vi "ExampleAll64.vi"() -> ()   [LabVIEW 2009]
uses:
  <userlib>/Untitled 5 Folder/user.lib/Shamrock64.llb/shamrock_flipperPort_typedef.ctl
  <userlib>/Untitled 5 Folder/user.lib/Shamrock64.llb/shamrock_lipperMirror_typedef.ctl
panel:
  in  "Device":i32 min=0 max=1
  in  "Set Device":bool
  in  "Tab Control":T1(tab)
  in  "Grating Offset":i32
  out "SetGratingOffset":string
  in  "Detector Offset":i32
  out "SetDetectorOffset":string
  out "WavelengthReset":string
  out "SetGrating":string
  in  "Grating":i32
  in  "Turret":i32
  out "SetTurret":string
  in  "SetGratingOffset":bool
  in  "SetDetectorOffset":bool
  in  "WavelengthReset":bool
  in  "SetGrating":bool
  in  "SetTurret":bool
  out "blaze":string
  out "Grating Offset":i32
  out "Detector Offset":i32
  out "offset":i32
  out "home":i32
  out "lines/mm":dbl format="%.2f"
  out "Grating":i32
  out "No Gratings":i32
  out "Turret":i32
  out "Is Grating ?":string
  out "GetGratingOffset":string
  out "GetDetectorOffset":string
  out "GetGratingInfo":string
  out "GetGrating":string
  out "GetNumberGratings":string
  out "GetTurret":string
  out "GratingIsPresent":string
  out "GetCalibration":string
  out "SetNumberPixels":string
  out "SetPixelWidth":string
  out "Max Dispersion":sgl
  out "Min Dispersion":sgl
  in  "Number Pixels":u32 caption="Numeric"
  in  "Pixel Width":sgl caption="Numeric" format="%_3g"
  out "GotoZeroOrder":string
  out "SetWavelength":string
  in  "Wavelength":dbl format="%.2f"
  in  "GoToZeroOrder":bool
  out "Max Wavelength":dbl format="%.2f"
  out "Min Wavelength":dbl format="%.2f"
  out "Is Wavelength ?":string
  out "WavelengthIsPresent":string
  out "GetWavelengthLimits":string
  out "At Zero Order ?":string
  out "AtZeroOrder":string
  out "Wavelength":dbl format="%.2f"
  in  "SetWavelength 2":bool
  out "GetWavelength":string
  in  "Reset Output Slit":bool
  in  "Reset Slit":bool
  out "ResetOutputSlit":string
  out "ResetSlit":string
  out "SetOutputSlit":string
  out "SetSlit":string
  in  "Output Slit Width":dbl format="%.2f"
  in  "SetOuputSlit":bool
  in  "Slit Width":dbl format="%.2f"
  in  "SetSlit 2":bool
  out "Output Slit width(mm)":dbl format="%.2f"
  out "Slit width (mm)":dbl format="%.2f"
  out "Is Output Slit ?":string
  out "Is Input Slit ?":string
  out "GetOutputSlit":string
  out "GetSlit":string
  out "OutputSlitIsPresent":string
  out "SlitIsPresent":string
  in  "Mode":i32
  in  "SetShutter":bool
  out "Is Mode Possible ?":string
  out "Shutter":i32
  out "Is Shutter ?":string
  out "SetShutter":string
  out "IsModePossible":string
  out "GetShutter":string
  out "ShutterIsPresent":string
  in  "Flipper Port":T2
  out "High":dbl format="%.2f"
  in  "FlipperReset":bool
  out "FlipperReset":string
  in  "SetPort":bool
  out "Low":dbl format="%.2f"
  out "Port":T2
  out "Is Flipper ?":string
  out "SetPort":string
  out "GetCCDLimits":string
  out "GetPort":string
  out "FlipperIsPresent":string
  out "GetFlipperMirror":string
  in  "FlipperSelect":bool
  in  "Flipper Mirror":T3
  in  "Filter info":string caption="String"
  out "Filter Info":string
  in  "SetFilterInfo":bool
  out "SetFilterInfo":string
  in  "Filter":i32
  in  "SetFilter":bool
  out "Filter":i32
  out "Is Filter ?":string
  out "SetFilter":string
  out "GetFilterInfo":string
  out "GetFilter":string
  out "FilterIsPresent":string
  in  "Line":i32
  out "Line 2":i32
  in  "State":i32
  in  "Set Accessory":bool
  out "Line 1":i32
  out "Is Accessory ?":string
  out "SetAccessory":string
  out "GetAccessory":string
  out "AccessoryIsPresent":string
  out "Initializing":bool
  in  "STOP if TRUE":bool
  out "Focal tilt":dbl format="%.2f"
  out "Angular deviation":dbl format="%.2f"
  out "Focal length":dbl format="%.2f"
  out "Serial Number":string
  out "No of devices":i32
  out "GetOpticalParameters":string
  out "GetSerialNumber":string
  out "GetNumberDevices":string
  out "Close":string
  out "Initialize":string
  # "INITIALIZATION"
  # "SDK RETURN VALUES"
  # "SHAMROCK PARAMETERS"
  # "ACTIONS"
  # "SDK RETURN VALUES"
  # "SHAMROCK PARAMETERS"
  # "ACTIONS"
  # "SDK RETURN VALUES"
  # "SHAMROCK PARAMETERS"
  # "ACTIONS"
  # "nm"
  # "Dispersion range"
  # "SDK RETURN VALUES"
  # "SHAMROCK PARAMETERS"
  # "ACTIONS"
  # "mm"
  # "mm"
  # "SDK RETURN VALUES"
  # "SHAMROCK PARAMETERS"
  # "ACTIONS"
  # "( 0:Closed / 1:Open )"
  # "SDK RETURN VALUES"
  # "SHAMROCK PARAMETERS"
  # "ACTIONS"
  # "SDK RETURN VALUES"
  # "SHAMROCK PARAMETERS"
  # "ACTIONS"
  # "SDK RETURN VALUES"
  # "SHAMROCK PARAMETERS"
  # "ACTIONS"
  # "line"
  # "to state"
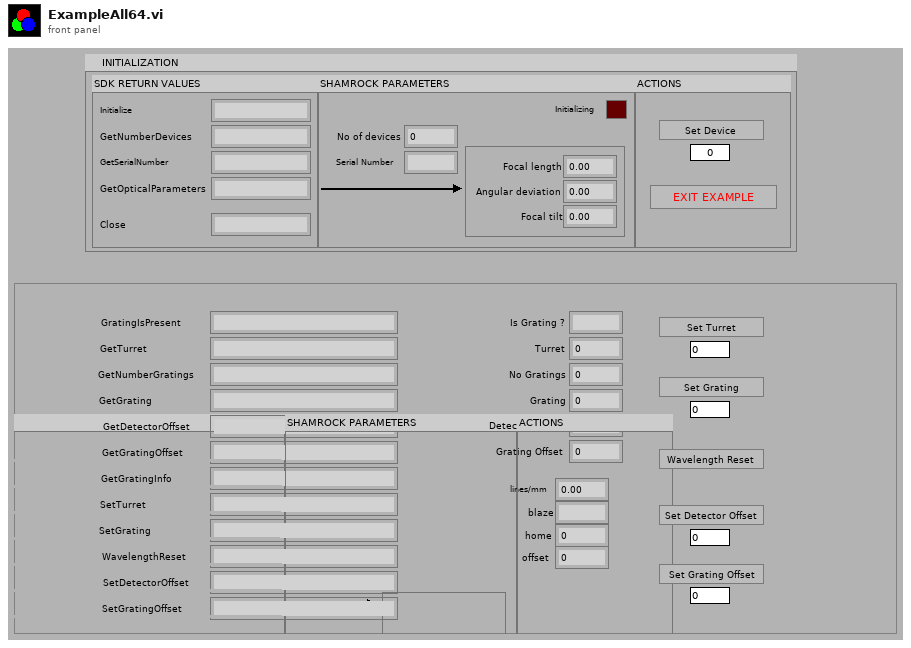
[diagram p1: front panel]
types:
  T1 = enum32{"GRATINGS", "WAVELENGTH", "INPUT & OUTPUT SLIT", "SHUTTER", "FLIPPER", "FILTER", "ACCESSORY"}
  T2 = typedef "shamrock_flipperPort_typedef.ctl" = enum32{"DIRECT PORT", "SIDE PORT"}
  T3 = typedef "shamrock_lipperMirror_typedef.ctl" = enum32{"Reserved (0)", "INPUT MIRROR", "OUTPUT MIRROR"}
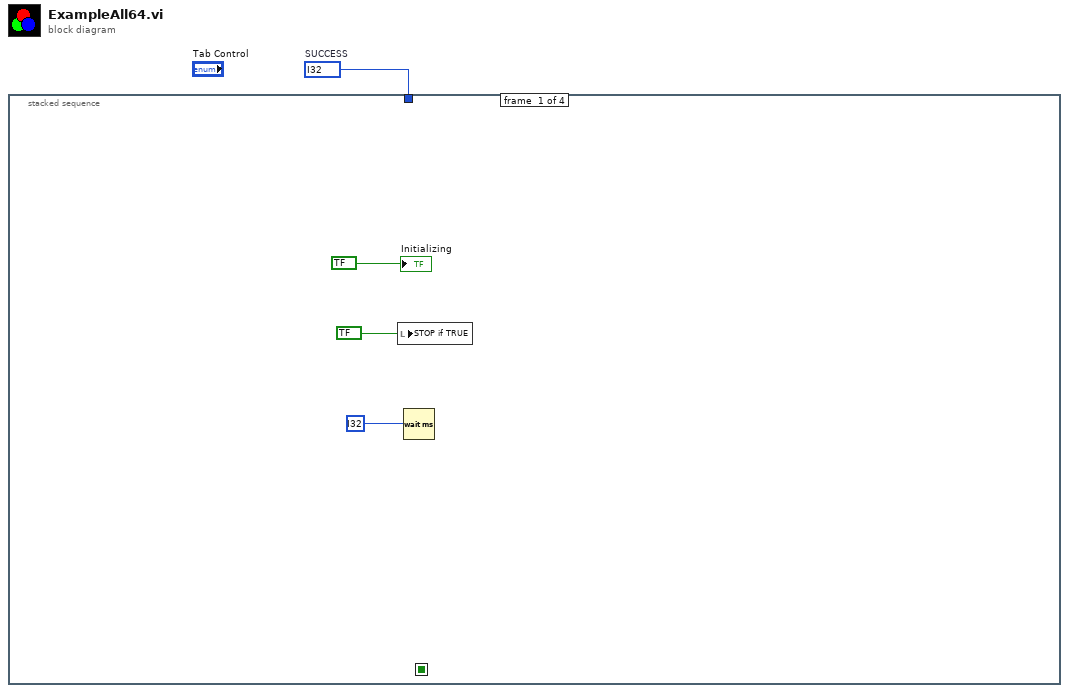
[diagram p0: block diagram]
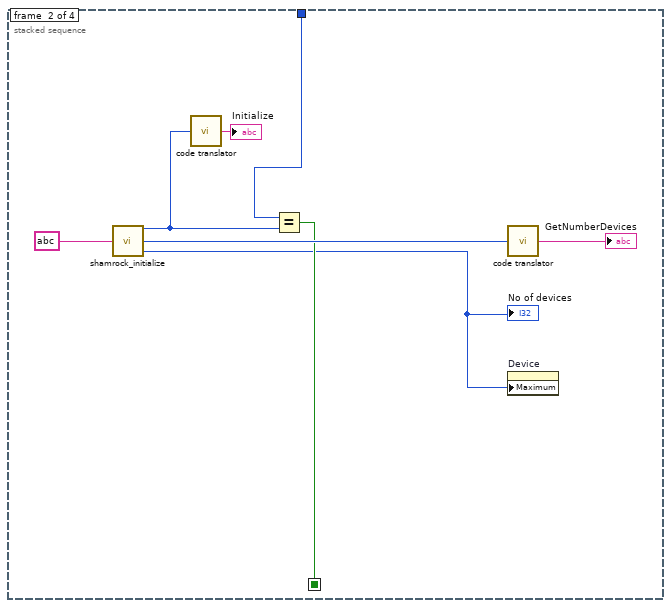
[diagram p2: hidden frame]
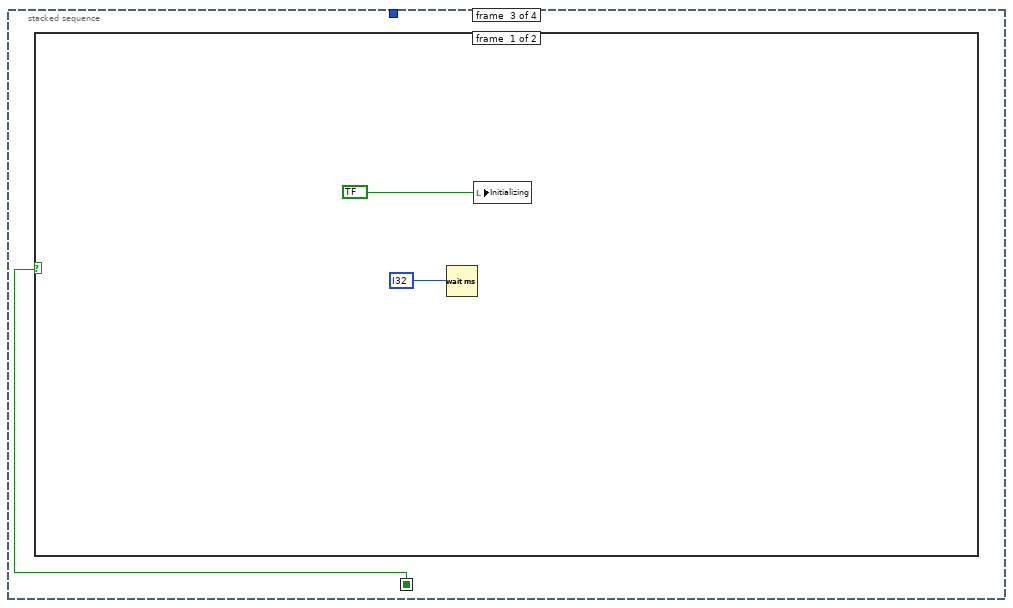
[diagram p3: hidden frame]
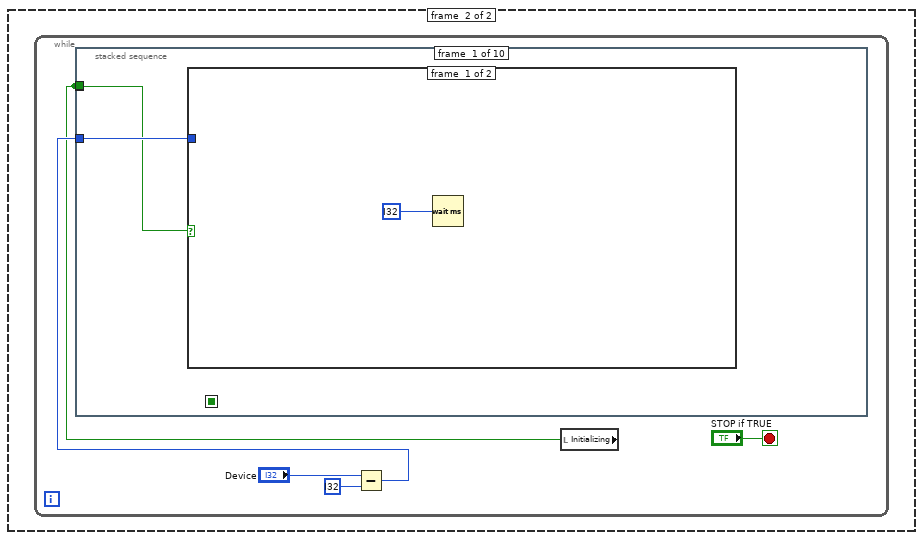
[diagram p4: hidden frame]
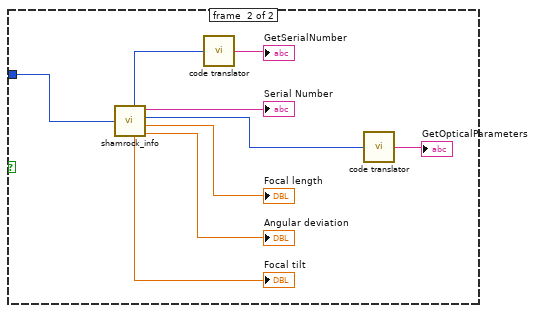
[diagram p5: hidden frame]
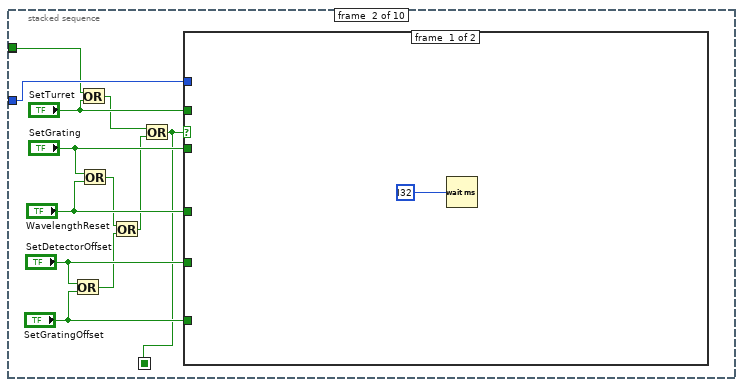
[diagram p6: hidden frame]
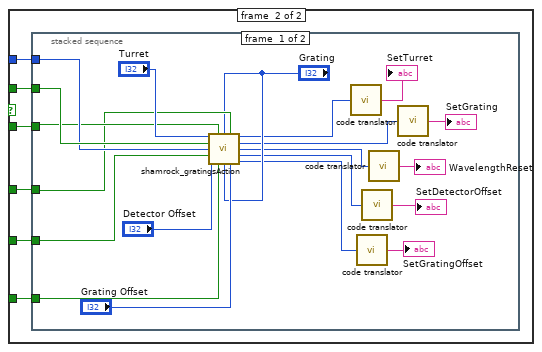
[diagram p7: hidden frame]
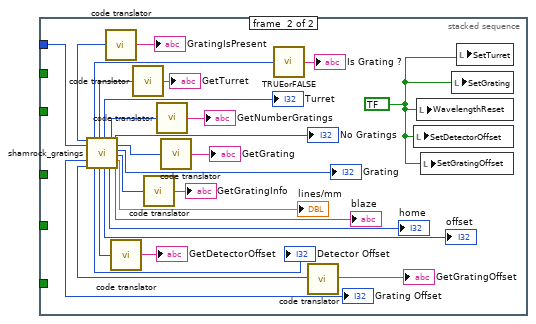
[diagram p8: hidden frame]
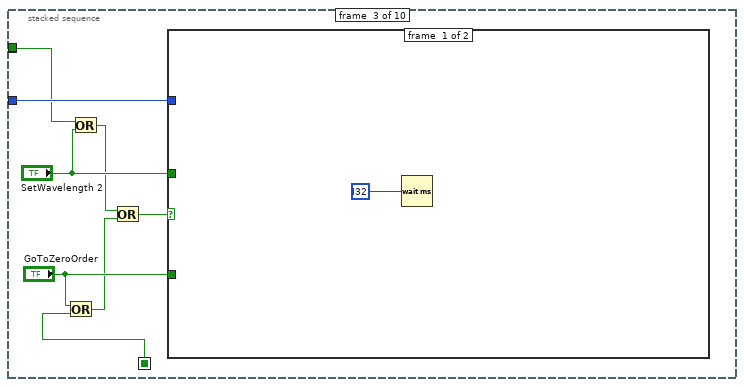
[diagram p9: hidden frame]
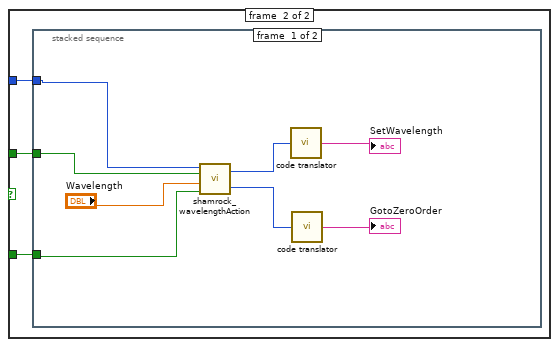
[diagram p10: hidden frame]
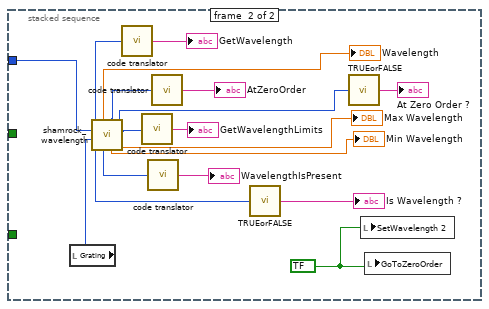
[diagram p11: hidden frame]
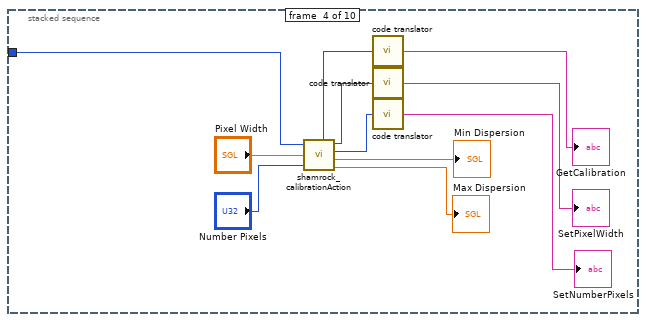
[diagram p12: hidden frame]
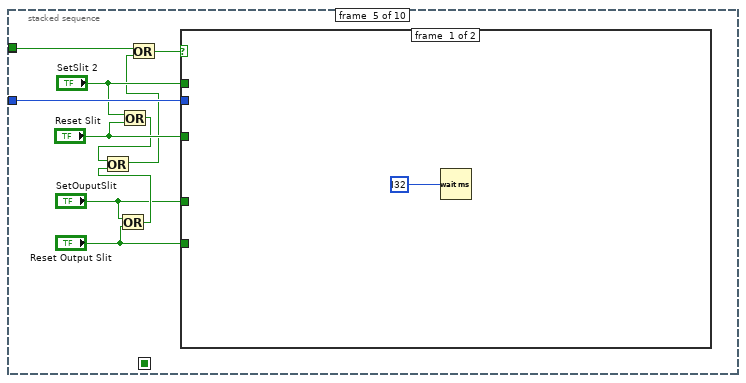
[diagram p13: hidden frame]
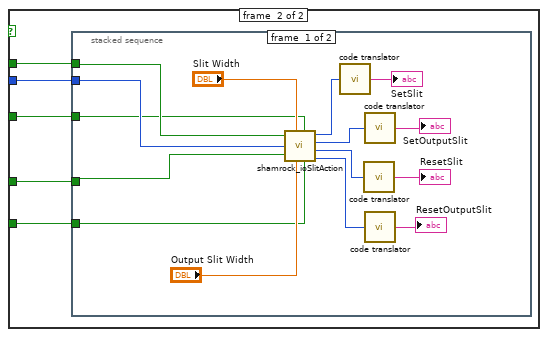
[diagram p14: hidden frame]
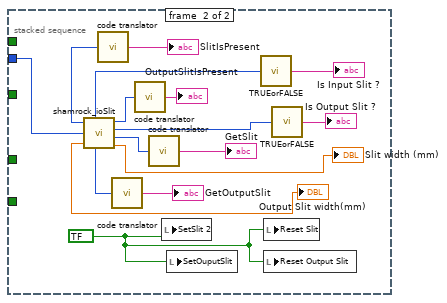
[diagram p15: hidden frame]
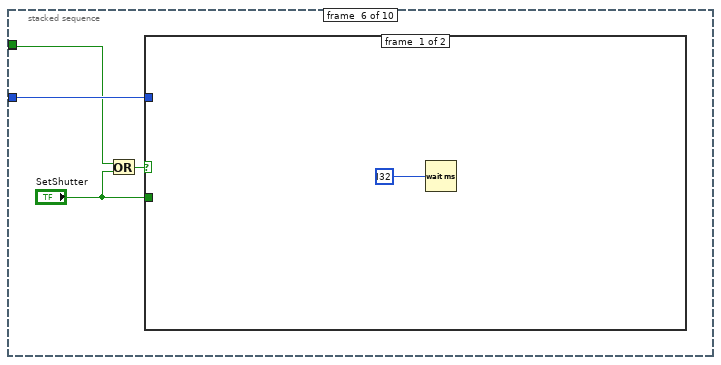
[diagram p16: hidden frame]
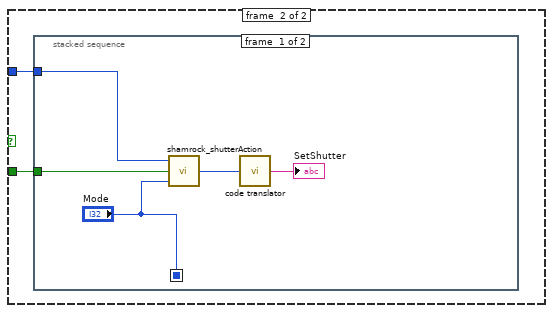
[diagram p17: hidden frame]
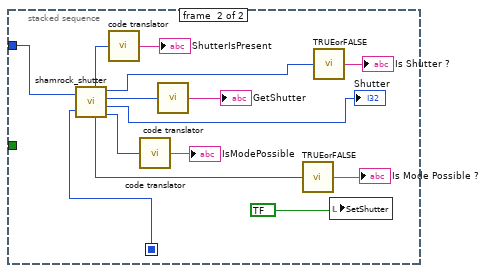
[diagram p18: hidden frame]
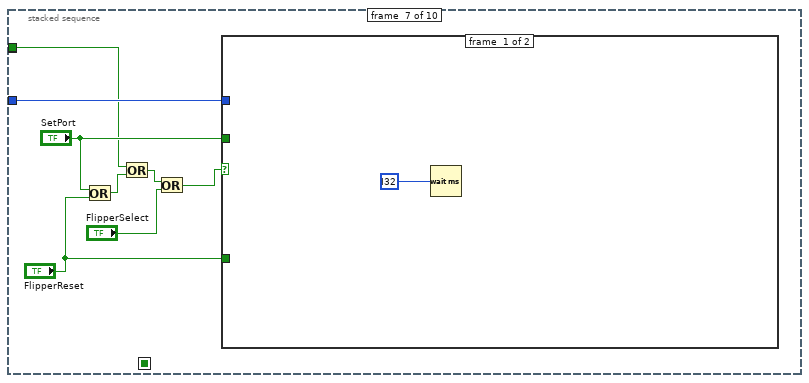
[diagram p19: hidden frame]
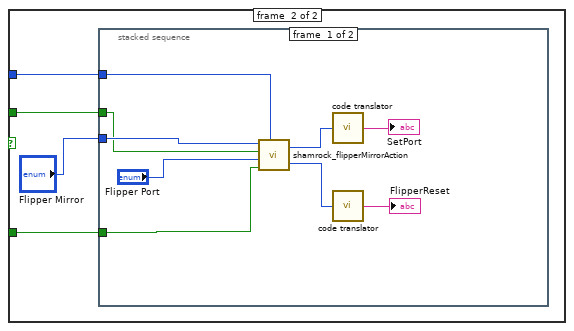
[diagram p20: hidden frame]
diagram:
  w1 = i32 ?  # SUCCESS
  n1 = stacked-sequence {
    seq-local: [_ w6 _ _] -> [_ _ w13 _]
    tunnel: w1 -> [_ w12 _ _]
    frame #0 {
      n2 = local write "STOP if TRUE"(bool ?) -> ()
      n3 = Wait (ms)(milliseconds to wait=i32 ?) -> ()  [unwired: 1 out]
      "Initializing" <- bool ?
    }
    frame #1 {
      n4 = call <userlib>:"shamrock_initialize.vi"("Initialization path"=string ?) -> ("Initialize"=w9:u32, "GetNumberDevices"=w8:u32, "No of devices"=w5:i32)
      "No of devices" <- w5
      n5 = call <userlib>:"code translator.vi"("Error code"=w9) -> ("Error description"=→"Initialize":string)
      n6 = Equal?(x=w12, y=w9) -> (x = y?=w6:bool)
      n7 = call <userlib>:"code translator.vi"("Error code"=w8) -> ("Error description"=→"GetNumberDevices":string)
      n8 = property on="Device" class="DigNum (strict)"("Maximum"=w5) -> ()  [unwired: 2 in, 2 out]
    }
    frame #2 {
      n9 = case shown="True" w13 {
        frame #0 {
          n10 = Wait (ms)(milliseconds to wait=i32 ?) -> ()  [unwired: 1 out]
          n11 = local write "Initializing"(bool ?) -> ()
        }
        frame #1 {
          n12 = while {
            stop <- "STOP if TRUE" stop-if-true
            n13 = Subtract(x="Device", y=i32 ?) -> (x-y=w19:i32)
            n14 = local read "Initializing"() -> (w16:bool)
            n15 = stacked-sequence {
              seq-local: [_ w33 _ _ _ _ _ _ _ _] -> [_ _ w105 _ _ _ _ _ _ _]
              tunnel: w19 -> [w22 w44 w106 w138 w157 w198 w228 w263 w292 _]
              tunnel: w16 -> [w21 w36 w102 _ w150 w195 _ w258 w289 _]
              tunnel: w16 -> [_ _ _ _ _ _ w224 _ _ _]
              frame #0 {
                n16 = case shown="True" w21 {
                  tunnel: w22 -> [_ w24]
                  frame #0 {
                    n17 = Wait (ms)(milliseconds to wait=i32 ?) -> ()  [unwired: 1 out]
                  }
                  frame #1 {
                    n18 = call <userlib>:"shamrock_info.vi"("Device No"=w24) -> ("GetSerialNumber"=w28:u32, "Focal tilt"=→"Focal tilt":sgl, "Serial Number"=→"Serial Number":string, "GetOpticalParameters"=w26:u32, "Focal length"=→"Focal length":sgl, "Angular deviation"=→"Angular deviation":sgl)
                    n19 = call <userlib>:"code translator.vi"("Error code"=w28) -> ("Error description"=→"GetSerialNumber":string)
                    n20 = call <userlib>:"code translator.vi"("Error code"=w26) -> ("Error description"=→"GetOpticalParameters":string)
                  }
                }
              }
              frame #1 {
                n21 = Or(x="SetDetectorOffset", y="SetGratingOffset") -> (x .or. y?=w38:bool)
                n22 = Or(x=w36, y="SetTurret") -> (x .or. y?=w35:bool)
                n23 = Or(x="SetGrating", y="WavelengthReset") -> (x .or. y?=w39:bool)
                n24 = Or(x=w39, y=w38) -> (x .or. y?=w34:bool)
                n25 = Or(x=w35, y=w34) -> (x .or. y?=w33:bool)
                n26 = case shown="True" w33 {
                  tunnel: w44 -> [_ w51]
                  tunnel: "SetDetectorOffset" -> [_ w50]
                  tunnel: "SetGratingOffset" -> [_ w49]
                  tunnel: "SetGrating" -> [_ w48]
                  tunnel: "WavelengthReset" -> [_ w47]
                  tunnel: "SetTurret" -> [_ w46]
                  frame #0 {
                    n27 = Wait (ms)(milliseconds to wait=i32 ?) -> ()  [unwired: 1 out]
                  }
                  frame #1 {
                    n28 = stacked-sequence {
                      tunnel: w46 -> [w70 _]
                      tunnel: w51 -> [w69 w89]
                      tunnel: w48 -> [w64 _]
                      tunnel: w47 -> [w63 _]
                      tunnel: w50 -> [w68 _]
                      tunnel: w49 -> [w66 _]
                      frame #0 {
                        n29 = call <userlib>:"shamrock_gratingsAction.vi"("WavelengthReset"=w63, "Grating Offset"="Grating Offset", 7:"Grating"="Grating", 8:"Grating"="Grating", "SetGrating"=w64, "SetGratingOffset"=w66, "Turret"="Turret", "SetTurret"=w70, "Device No"=w69, "SetDetectorOffset"=w68, "Detector Offset"="Detector Offset") -> ("SetTurret"=w61:u32, "SetGrating"=w59:u32, "WavelengthReset"=w56:u32, "SetDetectorOffset"=w54:u32, "SetGratingOffset"=w53:u32)
                        n30 = call <userlib>:"code translator.vi"("Error code"=w61) -> ("Error description"=→"SetTurret":string)
                        n31 = call <userlib>:"code translator.vi"("Error code"=w53) -> ("Error description"=→"SetGratingOffset":string)
                        n32 = call <userlib>:"code translator.vi"("Error code"=w54) -> ("Error description"=→"SetDetectorOffset":string)
                        n33 = call <userlib>:"code translator.vi"("Error code"=w56) -> ("Error description"=→"WavelengthReset":string)
                        n34 = call <userlib>:"code translator.vi"("Error code"=w59) -> ("Error description"=→"SetGrating":string)
                      }
                      frame #1 {
                        w98 = bool ?
                        n35 = call <userlib>:"shamrock_gratings.vi"("Device No"=w89) -> ("No Gratings"=→"No Gratings":i32, "GetNumberGratings"=w83:u32, "Turret"=→"Turret":i32, "GetTurret"=w85:u32, "0:FALSE / 1:TRUE"=w73:i32, "GratingIsPresent"=w87:u32, "GetGrating"=w81:u32, "Grating"=→"Grating":i32, "GetGratingInfo"=w79:u32, "lines/mm"=→"lines/mm":dbl, "Grating Offset"=→"Grating Offset":i32, "blaze"=→"blaze":string, "home"=→"home":i32, "offset"=→"offset":i32, "GetDetectorOffset"=w77:u32, "Detector Offset"=→"Detector Offset":i32, "GetGratingOffset"=w75:u32)  [unwired: 1 in, 1 out]
                        n36 = call <userlib>:"code translator.vi"("Error code"=w87) -> ("Error description"=→"GratingIsPresent":string)
                        n37 = call <userlib>:"code translator.vi"("Error code"=w77) -> ("Error description"=→"GetDetectorOffset":string)
                        n38 = call <userlib>:"code translator.vi"("Error code"=w85) -> ("Error description"=→"GetTurret":string)
                        n39 = call <userlib>:"code translator.vi"("Error code"=w79) -> ("Error description"=→"GetGratingInfo":string)
                        n40 = call <userlib>:"code translator.vi"("Error code"=w83) -> ("Error description"=→"GetNumberGratings":string)
                        n41 = call <userlib>:"code translator.vi"("Error code"=w81) -> ("Error description"=→"GetGrating":string)
                        n42 = call <userlib>:"TRUEorFALSE.vi"("bool number"=w73) -> ("String"=→"Is Grating ?":string)
                        n43 = call <userlib>:"code translator.vi"("Error code"=w75) -> ("Error description"=→"GetGratingOffset":string)
                        n44 = local write "SetDetectorOffset"(w98) -> ()
                        n45 = local write "WavelengthReset"(w98) -> ()
                        n46 = local write "SetGratingOffset"(w98) -> ()
                        n47 = local write "SetGrating"(w98) -> ()
                        n48 = local write "SetTurret"(w98) -> ()
                      }
                    }
                  }
                }
              }
              frame #2 {
                n49 = Or(x="GoToZeroOrder", y=w105) -> (x .or. y?=w100:bool)
                n50 = Or(x=w102, y="SetWavelength 2") -> (x .or. y?=w101:bool)
                n51 = Or(x=w101, y=w100) -> (x .or. y?=w99:bool)
                n52 = case shown="True" w99 {
                  tunnel: "SetWavelength 2" -> [_ w110]
                  tunnel: "GoToZeroOrder" -> [_ w109]
                  tunnel: w106 -> [_ w108]
                  frame #0 {
                    n53 = Wait (ms)(milliseconds to wait=i32 ?) -> ()  [unwired: 1 out]
                  }
                  frame #1 {
                    n54 = stacked-sequence {
                      tunnel: w110 -> [w116 _]
                      tunnel: w109 -> [w117 _]
                      tunnel: w108 -> [w115 w131]
                      frame #0 {
                        n55 = call <userlib>:"shamrock_wavelengthAction.vi"("GoToZeroOrder"=w117, "Wavelength"="Wavelength", "SetWavelength"=w116, "Device No"=w115) -> ("GotoZeroOrder"=w112:u32, "SetWavelength"=w114:u32)
                        n56 = call <userlib>:"code translator.vi"("Error code"=w114) -> ("Error description"=→"SetWavelength":string)
                        n57 = call <userlib>:"code translator.vi"("Error code"=w112) -> ("Error description"=→"GotoZeroOrder":string)
                      }
                      frame #1 {
                        w136 = bool ?
                        n58 = local read "Grating"() -> (w132:i32)
                        n59 = call <userlib>:"shamrock_wavelength.vi"("Grating No"=w132, "Device No"=w131) -> (0:"0:FALSE / 1:TRUE"=w120:i32, "WavelengthIsPresent"=w124:u32, "Min wl"=→"Min Wavelength":dbl, "Max wl"=→"Max Wavelength":dbl, "GetWavelengthLimits"=w126:u32, "GetWavelength"=w130:u32, "Wavelength"=→"Wavelength":dbl, "AtZeroOrder"=w128:u32, 10:"0:FALSE / 1:TRUE"=w122:i32)
                        n60 = call <userlib>:"code translator.vi"("Error code"=w130) -> ("Error description"=→"GetWavelength":string)
                        n61 = call <userlib>:"code translator.vi"("Error code"=w126) -> ("Error description"=→"GetWavelengthLimits":string)
                        n62 = call <userlib>:"code translator.vi"("Error code"=w124) -> ("Error description"=→"WavelengthIsPresent":string)
                        n63 = call <userlib>:"code translator.vi"("Error code"=w128) -> ("Error description"=→"AtZeroOrder":string)
                        n64 = call <userlib>:"TRUEorFALSE.vi"("bool number"=w120) -> ("String"=→"Is Wavelength ?":string)
                        n65 = call <userlib>:"TRUEorFALSE.vi"("bool number"=w122) -> ("String"=→"At Zero Order ?":string)
                        n66 = local write "SetWavelength 2"(w136) -> ()
                        n67 = local write "GoToZeroOrder"(w136) -> ()
                      }
                    }
                  }
                }
              }
              frame #3 {
                n68 = call <userlib>:"shamrock_calibrationAction.vi"("Device No"=w138, "Set Pixel Width"="Pixel Width", "Set Number Pixels"="Number Pixels") -> ("Set Pixel Width"=w145:u32, "Set Number Pixels"=w143:u32, "Wavelength First Pixel"=→"Min Dispersion":sgl, "Wavelength Last Pixel"=→"Max Dispersion":sgl, "GetCalibration"=w147:u32)
                n69 = call <userlib>:"code translator.vi"("Error code"=w147) -> ("Error description"=→"GetCalibration":string)
                n70 = call <userlib>:"code translator.vi"("Error code"=w145) -> ("Error description"=→"SetPixelWidth":string)
                n71 = call <userlib>:"code translator.vi"("Error code"=w143) -> ("Error description"=→"SetNumberPixels":string)
              }
              frame #4 {
                n72 = Or(x="SetOuputSlit", y="Reset Output Slit") -> (x .or. y?=w154:bool)
                n73 = Or(x="SetSlit 2", y="Reset Slit") -> (x .or. y?=w153:bool)
                n74 = Or(x=w153, y=w154) -> (x .or. y?=w152:bool)
                n75 = Or(x=w150, y=w152) -> (x .or. y?=w151:bool)
                n76 = case shown="True" w151 {
                  tunnel: w157 -> [_ w163]
                  tunnel: "SetSlit 2" -> [_ w162]
                  tunnel: "Reset Slit" -> [_ w161]
                  tunnel: "Reset Output Slit" -> [_ w160]
                  tunnel: "SetOuputSlit" -> [_ w159]
                  frame #0 {
                    n77 = Wait (ms)(milliseconds to wait=i32 ?) -> ()  [unwired: 1 out]
                  }
                  frame #1 {
                    n78 = stacked-sequence {
                      tunnel: w162 -> [w174 _]
                      tunnel: w160 -> [w173 _]
                      tunnel: w163 -> [w178 w191]
                      tunnel: w159 -> [w177 _]
                      tunnel: w161 -> [w172 _]
                      frame #0 {
                        n79 = call <userlib>:"shamrock_ioSlitAction.vi"("SetSlit"=w174, "Slit Width"="Slit Width", "Device No"=w178, "SetOuputSlit"=w177, "Output Slit Width"="Output Slit Width", "Reset Slit"=w172, "Reset Output Slit"=w173) -> ("SetSlit"=w171:u32, "SetOutputSlit"=w169:u32, "ResetSlit"=w167:u32, "ResetOutputSlit"=w164:u32)
                        n80 = call <userlib>:"code translator.vi"("Error code"=w171) -> ("Error description"=→"SetSlit":string)
                        n81 = call <userlib>:"code translator.vi"("Error code"=w167) -> ("Error description"=→"ResetSlit":string)
                        n82 = call <userlib>:"code translator.vi"("Error code"=w169) -> ("Error description"=→"SetOutputSlit":string)
                        n83 = call <userlib>:"code translator.vi"("Error code"=w164) -> ("Error description"=→"ResetOutputSlit":string)
                      }
                      frame #1 {
                        w194 = bool ?
                        n84 = call <userlib>:"shamrock_ioSlit.vi"("Device No"=w191) -> ("SlitIsPresent"=w190:u32, 1:"0:FALSE / 1:TRUE"=w182:i32, "Output Slit width(mm)"=→"Output Slit width(mm)":dbl, "GetOutputSlit"=w184:u32, "OutputSlitIsPresent"=w188:u32, 6:"0:FALSE / 1:TRUE"=w179:i32, "GetSlit"=w186:u32, "Slit width (mm)"=→"Slit width (mm)":dbl)
                        n85 = call <userlib>:"code translator.vi"("Error code"=w190) -> ("Error description"=→"SlitIsPresent":string)
                        n86 = call <userlib>:"code translator.vi"("Error code"=w184) -> ("Error description"=→"GetOutputSlit":string)
                        n87 = call <userlib>:"code translator.vi"("Error code"=w188) -> ("Error description"=→"OutputSlitIsPresent":string)
                        n88 = call <userlib>:"code translator.vi"("Error code"=w186) -> ("Error description"=→"GetSlit":string)
                        n89 = local write "SetSlit 2"(w194) -> ()
                        n90 = local write "SetOuputSlit"(w194) -> ()
                        n91 = call <userlib>:"TRUEorFALSE.vi"("bool number"=w182) -> ("String"=→"Is Input Slit ?":string)
                        n92 = local write "Reset Slit"(w194) -> ()
                        n93 = local write "Reset Output Slit"(w194) -> ()
                        n94 = call <userlib>:"TRUEorFALSE.vi"("bool number"=w179) -> ("String"=→"Is Output Slit ?":string)
                      }
                    }
                  }
                }
              }
              frame #5 {
                n95 = Or(x=w195, y="SetShutter") -> (x .or. y?=w196:bool)
                n96 = case shown="True" w196 {
                  tunnel: w198 -> [_ w201]
                  tunnel: "SetShutter" -> [_ w200]
                  frame #0 {
                    n97 = Wait (ms)(milliseconds to wait=i32 ?) -> ()  [unwired: 1 out]
                  }
                  frame #1 {
                    n98 = stacked-sequence {
                      seq-local: ["Mode" _] -> [_ w217]
                      tunnel: w201 -> [w204 w218]
                      tunnel: w200 -> [w205 _]
                      frame #0 {
                        n99 = call <userlib>:"shamrock_shutterAction.vi"("Mode"="Mode", "SetShutter"=w205, "Device No"=w204) -> ("SetShutter"=w203:u32)
                        n100 = call <userlib>:"code translator.vi"("Error code"=w203) -> ("Error description"=→"SetShutter":string)
                      }
                      frame #1 {
                        n101 = call <userlib>:"shamrock_shutter.vi"("Device No"=w218, "Mode"=w217) -> ("ShutterIsPresent"=w216:u32, 3:"0:FALSE / 1:TRUE"=w208:i32, 4:"0:FALSE / 1:TRUE"=w209:i32, "GetShutter"=w214:u32, "Shutter"=→"Shutter":i32, "IsModePossible"=w212:u32)
                        n102 = call <userlib>:"code translator.vi"("Error code"=w216) -> ("Error description"=→"ShutterIsPresent":string)
                        n103 = call <userlib>:"code translator.vi"("Error code"=w212) -> ("Error description"=→"IsModePossible":string)
                        n104 = call <userlib>:"code translator.vi"("Error code"=w214) -> ("Error description"=→"GetShutter":string)
                        n105 = call <userlib>:"TRUEorFALSE.vi"("bool number"=w208) -> ("String"=→"Is Mode Possible ?":string)
                        n106 = call <userlib>:"TRUEorFALSE.vi"("bool number"=w209) -> ("String"=→"Is Shutter ?":string)
                        n107 = local write "SetShutter"(bool ?) -> ()
                      }
                    }
                  }
                }
              }
              frame #6 {
                n108 = Or(x="SetPort", y="FlipperReset") -> (x .or. y?=w225:bool)
                n109 = Or(x=w224, y=w225) -> (x .or. y?=w223:bool)
                n110 = Or(x=w223, y="FlipperSelect") -> (x .or. y?=w221:bool)
                n111 = case shown="True" w221 {
                  tunnel: "SetPort" -> [_ w233]
                  tunnel: "FlipperReset" -> [_ w232]
                  tunnel: w228 -> [_ w231]
                  frame #0 {
                    n112 = Wait (ms)(milliseconds to wait=i32 ?) -> ()  [unwired: 1 out]
                  }
                  frame #1 {
                    n113 = stacked-sequence {
                      tunnel: w233 -> [w236 _]
                      tunnel: w232 -> [w235 _]
                      tunnel: w231 -> [w238 w252]
                      tunnel: "Flipper Mirror" -> [w237 w251]
                      frame #0 {
                        n114 = call <userlib>:"shamrock_flipperMirrorAction.vi"(0:w237, "SetPort"=w236, 2:"Flipper Port", "FlipperReset"=w235, "Device No"=w238) -> ("RC_SetPort"=w242:u32, "RC_FlipperReset"=w241:u32)
                        n115 = call <userlib>:"code translator.vi"("Error code"=w242) -> ("Error description"=→"SetPort":string)
                        n116 = call <userlib>:"code translator.vi"("Error code"=w241) -> ("Error description"=→"FlipperReset":string)
                      }
                      frame #1 {
                        w257 = bool ?
                        n117 = call <userlib>:"shamrock_flipperMirror.vi"("Flipper"=w251, "Device No"=w252) -> ("High"=→"High":dbl, "RC_GetCCDLimits"=w248:u32, "Low"=→"Low":dbl, "Flipper Port"=w243:T2, "RC_GetFlipperMirror"=w245:u32, "IsPresent"=w244:i32, "RC_FlipperIsPresent"=w247:u32)
                        "Port" <- w243
                        n118 = call <userlib>:"code translator.vi"("Error code"=w245) -> ("Error description"=→"GetFlipperMirror":string)
                        n119 = call <userlib>:"code translator.vi"("Error code"=w248) -> ("Error description"=→"GetCCDLimits":string)
                        n120 = call <userlib>:"code translator.vi"("Error code"=w247) -> ("Error description"=→"FlipperIsPresent":string)
                        n121 = call <userlib>:"code translator.vi"("Error code"=w243) -> ("Error description"=→"GetPort":string)
                        n122 = local write "SetPort"(w257) -> ()
                        n123 = local write "FlipperReset"(w257) -> ()
                        n124 = call <userlib>:"TRUEorFALSE.vi"("bool number"=w244) -> ("String"=→"Is Flipper ?":string)
                      }
                    }
                  }
                }
              }
              frame #7 {
                n125 = Or(x="SetFilter", y="SetFilterInfo") -> (x .or. y?=w260:bool)
                n126 = Or(x=w258, y=w260) -> (x .or. y?=w259:bool)
                n127 = case shown="True" w259 {
                  tunnel: w263 -> [_ w267]
                  tunnel: "SetFilter" -> [_ w266]
                  tunnel: "SetFilterInfo" -> [_ w265]
                  frame #0 {
                    n128 = Wait (ms)(milliseconds to wait=i32 ?) -> ()  [unwired: 1 out]
                  }
                  frame #1 {
                    n129 = stacked-sequence {
                      tunnel: w267 -> [w273 w285]
                      tunnel: w266 -> [w276 _]
                      tunnel: w265 -> [w275 _]
                      frame #0 {
                        n130 = call <userlib>:"shamrock_filterAction.vi"("Filter info"="Filter info", "Device No"=w273, 4:"Filter"="Filter", "SetFilterInfo"=w275, 6:"Filter"="Filter", "SetFilter"=w276) -> ("SetFilterInfo"=w268:u32, "SetFilter"=w271:u32)
                        n131 = call <userlib>:"code translator.vi"("Error code"=w271) -> ("Error description"=→"SetFilter":string)
                        n132 = call <userlib>:"code translator.vi"("Error code"=w268) -> ("Error description"=→"SetFilterInfo":string)
                      }
                      frame #1 {
                        w288 = bool ?
                        n133 = call <userlib>:"shamrock_filter.vi"("Device No"=w285) -> ("FilterIsPresent"=w284:u32, "Filter Info"=→"Filter Info":string, "0:FALSE / 1:TRUE"=w277:i32, "GetFilter"=w282:u32, "Filter"=→"Filter":i32, "GetFilterInfo"=w280:u32)
                        n134 = call <userlib>:"code translator.vi"("Error code"=w284) -> ("Error description"=→"FilterIsPresent":string)
                        n135 = call <userlib>:"code translator.vi"("Error code"=w280) -> ("Error description"=→"GetFilterInfo":string)
                        n136 = call <userlib>:"code translator.vi"("Error code"=w282) -> ("Error description"=→"GetFilter":string)
                        n137 = call <userlib>:"TRUEorFALSE.vi"("bool number"=w277) -> ("String"=→"Is Filter ?":string)
                        n138 = local write "SetFilter"(w288) -> ()
                        n139 = local write "SetFilterInfo"(w288) -> ()
                      }
                    }
                  }
                }
              }
              frame #8 {
                n140 = Or(x=w289, y="Set Accessory") -> (x .or. y?=w291:bool)
                n141 = case shown="True" w291 {
                  tunnel: w292 -> [_ w295]
                  tunnel: "Set Accessory" -> [_ w294]
                  frame #0 {
                    n142 = Wait (ms)(milliseconds to wait=i32 ?) -> ()  [unwired: 1 out]
                  }
                  frame #1 {
                    n143 = stacked-sequence {
                      tunnel: w295 -> [w298 w308]
                      tunnel: w294 -> [w301 _]
                      frame #0 {
                        n144 = call <userlib>:"shamrock_accessoryAction.vi"("State"="State", "Line"="Line", "Set Accessory"=w301, "Device No"=w298) -> ("SetAccessory"=w297:u32)
                        n145 = call <userlib>:"code translator.vi"("Error code"=w297) -> ("Error description"=→"SetAccessory":string)
                      }
                      frame #1 {
                        n146 = call <userlib>:"shamrock_accessory.vi"("Device No"=w308) -> ("Line 2"=→"Line 2":i32, "Line 1"=→"Line 1":i32, "Line 1 & Line 2"=w305:u32, "0:FALSE / 1:TRUE"=w303:i32, "AccessoryIsPresent"=w306:u32)
                        n147 = call <userlib>:"code translator.vi"("Error code"=w306) -> ("Error description"=→"AccessoryIsPresent":string)
                        n148 = call <userlib>:"code translator.vi"("Error code"=w305) -> ("Error description"=→"GetAccessory":string)
                        n149 = call <userlib>:"TRUEorFALSE.vi"("bool number"=w303) -> ("String"=→"Is Accessory ?":string)
                        n150 = local write "Set Accessory"(bool ?) -> ()
                      }
                    }
                  }
                }
              }
              frame #9 {
                n151 = case shown="True" "Set Device" {
                  frame #0 {
                    n152 = local write "Initializing"(bool ?) -> ()
                  }
                  frame #1 {
                    n153 = stacked-sequence {
                      frame #0 {
                        n154 = local write "Initializing"(bool ?) -> ()
                      }
                      frame #1 {
                        n155 = local write "Set Device"(bool ?) -> ()
                      }
                    }
                  }
                }
              }
            }
          }
        }
      }
    }
    frame #3 {
      n156 = call <userlib>:"shamrock_close.vi"() -> ("Close"=w317:u32)
      n157 = call <userlib>:"code translator.vi"("Error code"=w317) -> ("Error description"=→"Close":string)
    }
  }
